vi "X_2.66_COOLPROP.vi"() -> ()   [LabVIEW 2022 SP3]
uses:
  Coolprop_64bit/CoolProp_advanced.llb/FluidCommon.ctl
  Coolprop_64bit/CoolProp_advanced.llb/FluidOfInterest.ctl
  Coolprop_64bit/Coolprop_lib.lvlib
panel:
  out "Data 4 Specifik volimen":dbl
  out "Data 3 Specifik volimen":dbl
  out "Data 2 Specifik volimen":dbl
  out "Data 1 Specifik volimen":dbl
  out "Data 4 Volume L":dbl
  out "Data 4 Volume m^3":dbl
  out "Data 3 Volume L":dbl
  out "Data 3 Volume m^3":dbl
  out "Data 2 Volume L":dbl
  out "Data 2 Volume m^3":dbl
  out "Data 1 Volume L":dbl
  out "Data 1 Volume m^3":dbl
  out "Data 4":T1
  out "Data 3":T1
  out "Data 2":T1
  out "Data 1":T1
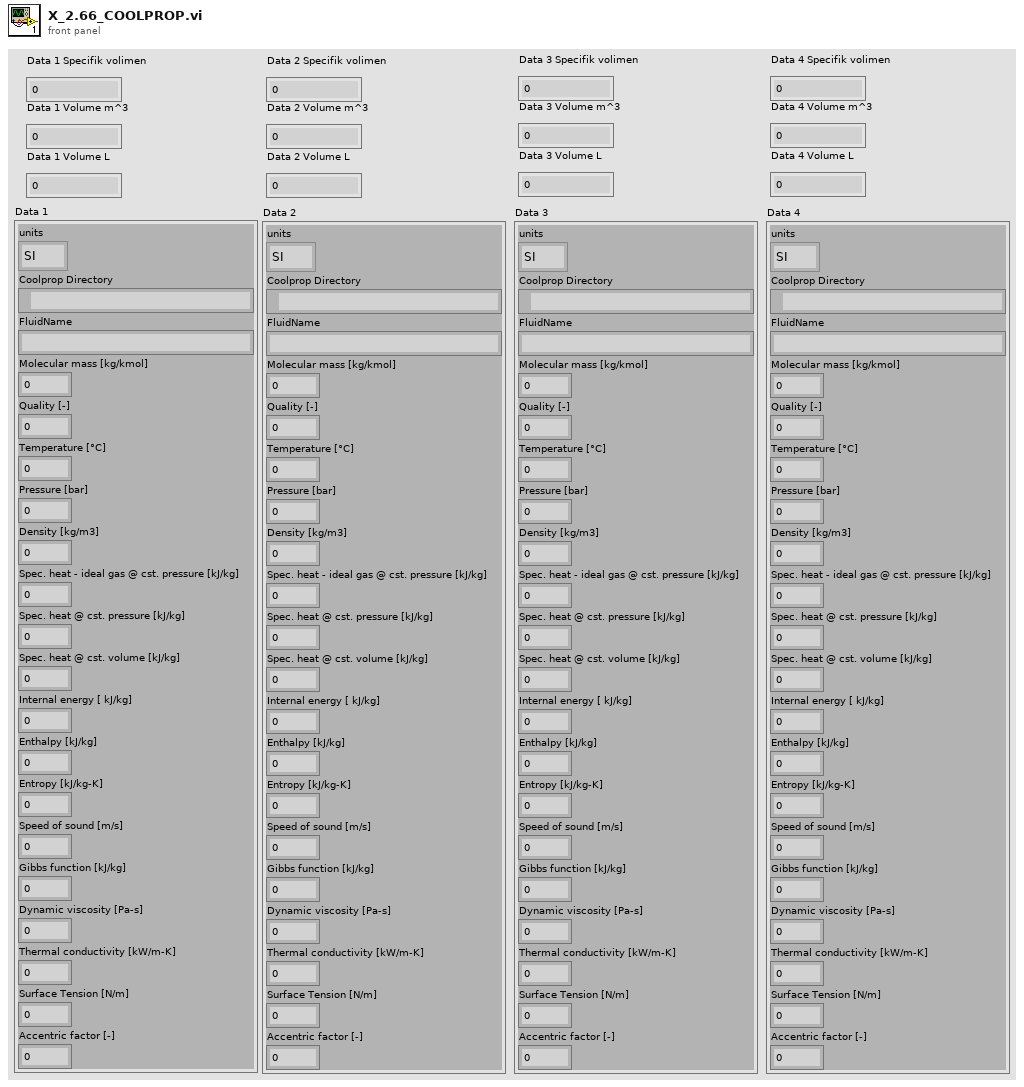
[diagram p1: front panel]
types:
  T1 = typedef "Coolprop_lib.lvlib/FluidCommon.ctl" = cluster{"units":enum16{"SI", "IP"}, "Coolprop Directory":path, "FluidName":string, "Molecular mass [kg/kmol]":dbl, "Quality [-]":dbl, "Temperature [°C]":dbl, "Pressure [bar]":dbl, "Density [kg/m3]":dbl, "Spec. heat - ideal gas @ cst. pressure [kJ/kg]":dbl, "Spec. heat @ cst. pressure [kJ/kg]":dbl, "Spec. heat @ cst. volume [kJ/kg]":dbl, "Internal energy [ kJ/kg]":dbl, "Enthalpy [kJ/kg]":dbl, "Entropy [kJ/kg-K]":dbl, "Speed of sound [m/s]":dbl, "Gibbs function [kJ/kg]":dbl, "Dynamic viscosity [Pa-s]":dbl, "Thermal conductivity [kW/m-K]":dbl, "Surface Tension [N/m]":dbl, "Accentric factor [-]":dbl}
  T2 = enum16{"0", "TP", "TD", "PD", "TQ", "PQ", "HP", "SP", "SH"}
  T3 = typedef "Coolprop_lib.lvlib/FluidOfInterest.ctl" = string
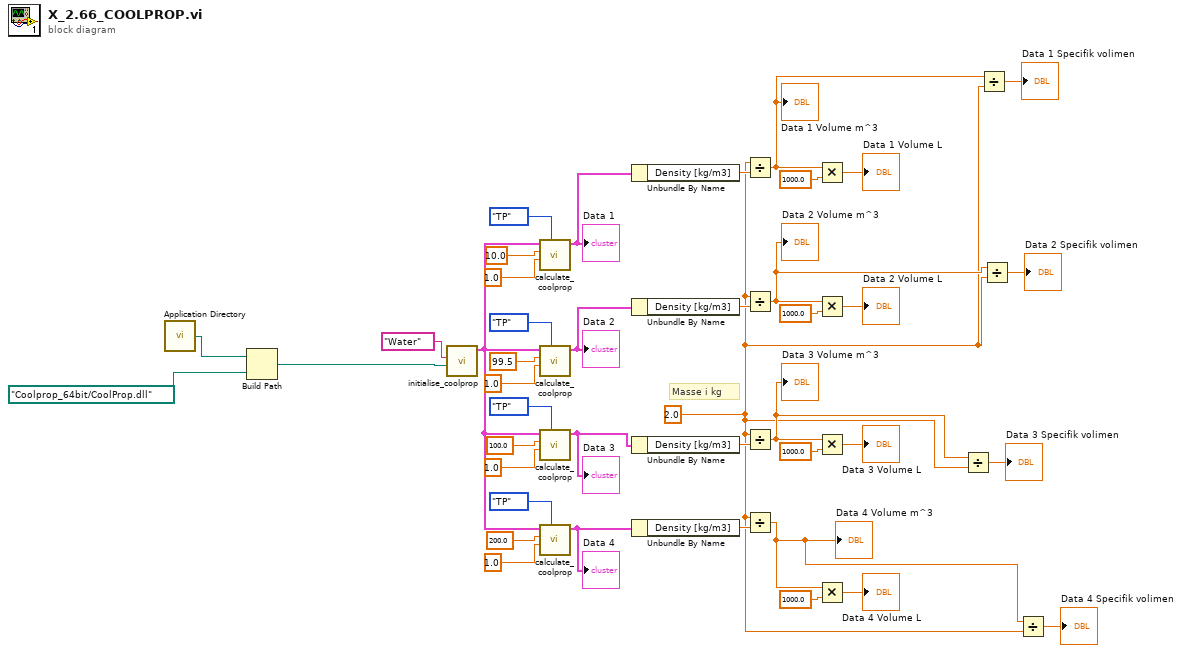
[diagram p0: block diagram]
diagram:
  w4 = 2.0
  # "Masse i kg"
  n1 = call <vilib>:"Application Directory.vi"() -> ("Application Directory"=w3:path)
  n2 = Build Path(base path=w3, name or relative path=path "Coolprop_64bit/CoolProp.dll") -> (appended path=w1:path)
  n3 = call "initialise_coolprop.vi"("Path to CoolProp.dll"=w1, "FluidOfInterest"=T3 "Water") -> ("Common Out"=w29:T1)  [unwired: 7 in, 2 out]
  n4 = call "calculate_coolprop.vi"("InputCode"=T2."TP", "Input_2"=1.0, "Input_1"=10.0, "Common In"=w29) -> ("Common Out"=w28:T1)  [unwired: 3 in, 1 out]
  "Data 1" <- w28
  n5 = call "calculate_coolprop.vi"("InputCode"=T2."TP", "Input_2"=1.0, "Input_1"=99.5, "Common In"=w29) -> ("Common Out"=w24:T1)  [unwired: 3 in, 1 out]
  "Data 2" <- w24
  n6 = call "calculate_coolprop.vi"("InputCode"=T2."TP", "Input_2"=1.0, "Input_1"=100.0, "Common In"=w29) -> ("Common Out"=w23:T1)  [unwired: 3 in, 1 out]
  "Data 3" <- w23
  n7 = call "calculate_coolprop.vi"("InputCode"=T2."TP", "Input_2"=1.0, "Input_1"=200.0, "Common In"=w29) -> ("Common Out"=w22:T1)  [unwired: 3 in, 1 out]
  "Data 4" <- w22
  n8 = Unbundle By Name(w28) -> ("Density [kg/m3]"=w27:dbl)
  n9 = Unbundle By Name(w24) -> ("Density [kg/m3]"=w15:dbl)
  n10 = Unbundle By Name(w23) -> ("Density [kg/m3]"=w14:dbl)
  n11 = Unbundle By Name(w22) -> ("Density [kg/m3]"=w13:dbl)
  n12 = Divide(x=w4, y=w27) -> (x/y=w12:dbl)
  "Data 1 Volume m^3" <- w12
  n13 = Divide(x=w4, y=w15) -> (x/y=w7:dbl)
  "Data 2 Volume m^3" <- w7
  n14 = Divide(x=w4, y=w14) -> (x/y=w6:dbl)
  "Data 3 Volume m^3" <- w6
  n15 = Divide(x=w4, y=w13) -> (x/y=w5:dbl)
  "Data 4 Volume m^3" <- w5
  n16 = Multiply(x=w12, y=1000.0) -> (x*y=→"Data 1 Volume L":dbl)
  n17 = Multiply(x=w7, y=1000.0) -> (x*y=→"Data 2 Volume L":dbl)
  n18 = Multiply(x=w6, y=1000.0) -> (x*y=→"Data 3 Volume L":dbl)
  n19 = Multiply(x=w5, y=1000.0) -> (x*y=→"Data 4 Volume L":dbl)
  n20 = Divide(x=w6, y=w4) -> (x/y=→"Data 3 Specifik volimen":dbl)
  n21 = Divide(x=w12, y=w4) -> (x/y=→"Data 1 Specifik volimen":dbl)
  n22 = Divide(x=w7, y=w4) -> (x/y=→"Data 2 Specifik volimen":dbl)
  n23 = Divide(x=w5, y=w4) -> (x/y=→"Data 4 Specifik volimen":dbl)
